vi "Write Output.vi"(8 "error in":errorcluster, 9 "Output Select":i32, 10 "Value":bool, 11 "PIOD in":refnum<class "PIOD.lvclass">) -> (0 "error out":errorcluster, 3 "PIOD out":refnum<class "PIOD.lvclass">)   [LabVIEW 2018, in "PIOD.lvlib" / "PIOD.lvclass"]
uses:
  PIOD.lvclass
  builds/PLC.lvlibp/PLC.lvclass
  C:/Users/Ron.Dexter.LUMINARTECH/Desktop/builds/PLC.lvlibp/PLC.lvclass
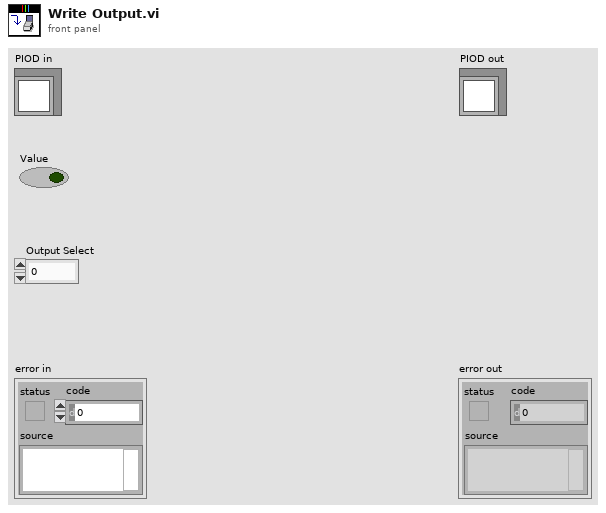
[diagram p1: front panel]
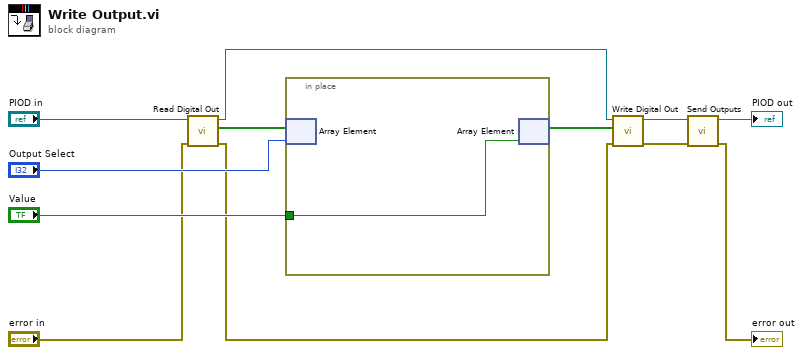
[diagram p0: block diagram]
diagram:
  n1 = call "Read Digital Out.vi"("error in"="error in", "PLC in"="PIOD in") -> ("error out"=w2:errorcluster, "Digital Out"=w8:bool[], "PLC out"=w5:refnum<class "PIOD.lvclass">)  [unwired: 7 in]
  n2 = in-place {
    in-place-border: "Value" -> [w13]
    n3 = in-place-array #1(w8, "Output Select") -> ()  [unwired: 1 out]
    n4 = in-place-array #1(w13) -> (w7:bool[])  [unwired: 1 out]
  }
  n5 = call "Write Digital Out.vi"("error in (no error)"=w2, "Digital Out"=w7, "PLC in"=w5) -> ("error out"=w1:errorcluster, "PLC out"=w6:refnum<class "PIOD.lvclass">)  [unwired: 7 in]
  n6 = call "Send Outputs.vi"("error in"=w1, "PIOD in"=w6) -> ("error out"=→"error out":errorcluster, "PIOD out"=→"PIOD out":refnum<class "PIOD.lvclass">)  [unwired: 8 in]
